vi "Acquire Data_RT.vi"(7 "Total Buffer Size":i32, 8 "error in (no error)":errorcluster, 9 "rt fifo":refnum<k33>, 10 "Acquisition and Logging Configuration":T1={"Data Rate"=1, "Samples per Read"=0, "Number of Reads to Save"=0, "Data File Name"="", "TDMS Properties"=[], "Number of Channels"=4, "Channel Scale Array"=[0.0, 0.0, 0.0, 0.0, 1.0, 1.0, 1.0, 1.0], "Channel Names"=[], "Trigger - RMS Value"=0.0, "Trigger - Channel"=0, "Trigger - Time (Minute)"=0} {"Data Rate" items=["51.200 kS/s (NI 9234)"=1, "25.600 kS/s (NI 9234)"=2, "17.067 kS/s (NI 9234)"=3, "12.800 kS/s (NI 9234)"=4, "10.240 kS/s (NI 9234)"=5, "8.533 kS/s (NI 9234)"=6, "7.314 kS/s (NI 9234)"=7, "6.400 kS/s (NI 9234)"=8, "5.689 kS/s (NI 9234)"=9, "5.120 kS/s (NI 9234)"=10, "4.654 kS/s (NI 9234)"=11, "4.267 kS/s (NI 9234)"=12, "3.938 kS/s (NI 9234)"=13, "3.657 kS/s (NI 9234)"=14, "3.413 kS/s (NI 9234)"=15, "3.200 kS/s (NI 9234)"=16, "3.012 kS/s (NI 9234)"=17, "2.845 kS/s (NI 9234)"=18, "2.695 kS/s (NI 9234)"=19, "2.560 kS/s (NI 9234)"=20, "2.438 kS/s (NI 9234)"=21, "2.328 kS/s (NI 9234)"=22, "2.226 kS/s (NI 9234)"=23, "2.133 kS/s (NI 9234)"=24, "2.048 kS/s (NI 9234)"=25, "1.969 kS/s (NI 9234)"=26, "1.896 kS/s (NI 9234)"=27, "1.829 kS/s (NI 9234)"=28, "1.765 kS/s (NI 9234)"=29, "1.707 kS/s (NI 9234)"=30, "1.652 kS/s (NI 9234)"=31]}, 11 "FPGA VI Reference":T4) -> (0 "error out":errorcluster, 2 "dup Acquisition and Logging Configuration":T1={"Data Rate"=1, "Samples per Read"=0, "Number of Reads to Save"=0, "Data File Name"="", "TDMS Properties"=[], "Number of Channels"=4, "Channel Scale Array"=[0.0, 0.0, 0.0, 0.0, 1.0, 1.0, 1.0, 1.0], "Channel Names"=[], "Trigger - RMS Value"=0.0, "Trigger - Channel"=0, "Trigger - Time (Minute)"=0} {"Data Rate" items=["51.200 kS/s (NI 9234)"=1, "25.600 kS/s (NI 9234)"=2, "17.067 kS/s (NI 9234)"=3, "12.800 kS/s (NI 9234)"=4, "10.240 kS/s (NI 9234)"=5, "8.533 kS/s (NI 9234)"=6, "7.314 kS/s (NI 9234)"=7, "6.400 kS/s (NI 9234)"=8, "5.689 kS/s (NI 9234)"=9, "5.120 kS/s (NI 9234)"=10, "4.654 kS/s (NI 9234)"=11, "4.267 kS/s (NI 9234)"=12, "3.938 kS/s (NI 9234)"=13, "3.657 kS/s (NI 9234)"=14, "3.413 kS/s (NI 9234)"=15, "3.200 kS/s (NI 9234)"=16, "3.012 kS/s (NI 9234)"=17, "2.845 kS/s (NI 9234)"=18, "2.695 kS/s (NI 9234)"=19, "2.560 kS/s (NI 9234)"=20, "2.438 kS/s (NI 9234)"=21, "2.328 kS/s (NI 9234)"=22, "2.226 kS/s (NI 9234)"=23, "2.133 kS/s (NI 9234)"=24, "2.048 kS/s (NI 9234)"=25, "1.969 kS/s (NI 9234)"=26, "1.896 kS/s (NI 9234)"=27, "1.829 kS/s (NI 9234)"=28, "1.765 kS/s (NI 9234)"=29, "1.707 kS/s (NI 9234)"=30, "1.652 kS/s (NI 9234)"=31]}, 3 "rt fifo out":refnum<k33>)   [LabVIEW 2015]
doc: "Reads waveform data from the DMA FIFO."
uses:
  controls/FPGA VI Reference.ctl
  controls/Acquisition and Logging Configuration.ctl
  <vilib>/LabVIEW Targets/FPGA/cRIO/shared/nicrio_ModuleControls/nicrio_cRIO-9234_DataRatesRing2.ctl
  controls/TDMS Properties.ctl
  <vilib>/Platform/TimedLoop/XDataNode/timing_clust.ctl
  <vilib>/Platform/TimedLoop/XDataNode/nitl_modes.ctl
  <vilib>/Platform/TimedLoop/XDataNode/wakeup.ctl
  <vilib>/Utility/error.llb/Error Cluster From Error Code.vi
  <vilib>/rvi/errors/niLvFpgaAdjustHostInterfaceError.vi
  Globals/Global - Monitoring Variables.vi
  <vilib>/rvi/interface/nirviReadWriteControl/nirviReadWriteControl.xnode
  <vilib>/rvi/interface/nirviMethod/nirviMethod.xnode
  <vilib>/Platform/TimedLoop/XDataNode/XDataNode.xnode
  NiFpgaLv.dll
  <vilib>/rvi/interface/Simulation/niFpgaSimulationCallBeginRW.vi
  <vilib>/FPGAPlugInAG/Dynamic/niLvFpga_ReadFifo_Dynamic.vi
  <vilib>/rvi/errors/niLvFpgaMergeErrorWithErrorCode.vi
  <vilib>/Platform/TimedLoop/XDataNode/XDNodeRunTimeDep.lvlib
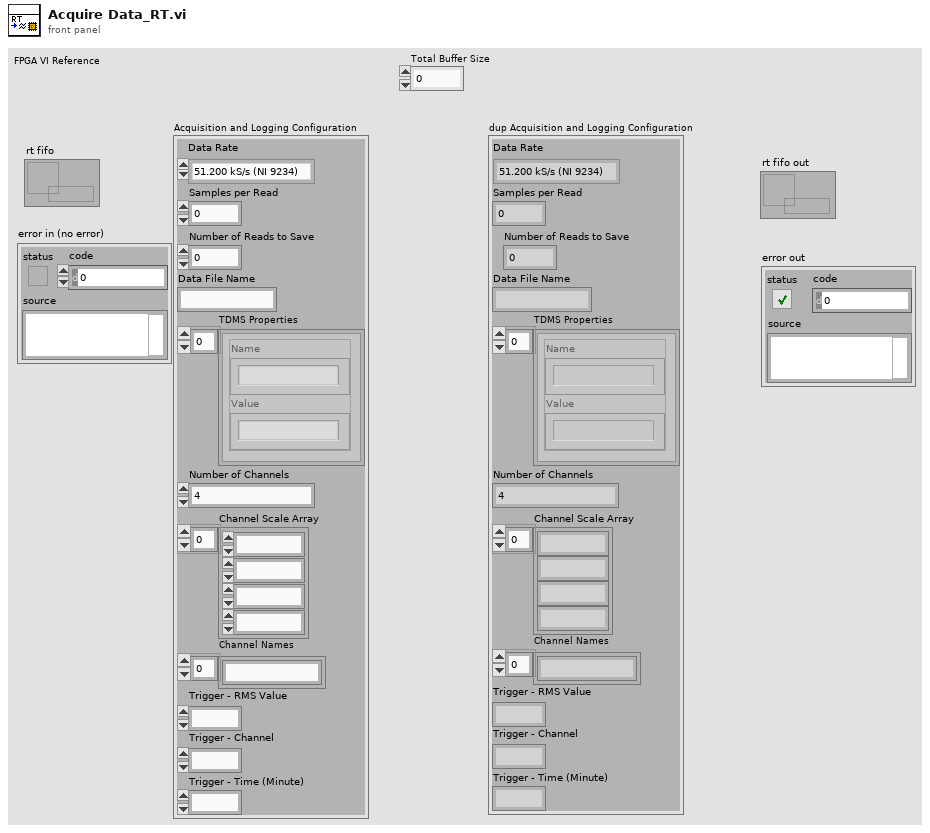
[diagram p1: front panel]
types:
  T1 = typedef "Acquisition and Logging Configuration.ctl" = cluster{"Data Rate":T2, "Samples per Read":i32, "Number of Reads to Save":i32, "Data File Name":string, "TDMS Properties":T3[], "Number of Channels":i32, "Channel Scale Array":fxp<+,24,12>[], "Channel Names":string[], "Trigger - RMS Value":dbl, "Trigger - Channel":i32, "Trigger - Time (Minute)":i32}
  T2 = typedef "nicrio_cRIO-9234_DataRatesRing2.ctl" = u8
  T3 = typedef "TDMS Properties.ctl" = cluster{"Name":string, "Value":string}
  T4 = typedef "FPGA VI Reference.ctl" = refnum<k20>
  T5 = typedef "XDNodeRunTimeDep.lvlib/timing_clust.ctl" = cluster{"Expected End [f-1]":u64, "Actual End [f-1]":u64, "Finished Late? [f-1]":bool, "Expected End [i-1]":u64, "Actual End [i-1]":u64, "Finished Late? [i-1]":bool, "Expected Start [i]":u64, "Actual Start [i]":u64, "Expected Start [f]":u64, "Actual Start [f]":u64, "Source Name":string, "Structure Name":string, "Period":i64, "Deadline":i64, "Offset":i64, "Start":i64, "Priority":i32, "Timeout":i32, "Mode":T6, "Wakeup Reason":T7, "Error":errorcluster, "Source Type":string, "Secondary Source Type":string, "Global End Time":u64, "Global Start Time":u64, "Frame Duration":u64, "Iteration Duration":u64, "Assigned CPU":i32, "I/O Scan Engine Mode":u32}
  T6 = typedef "XDNodeRunTimeDep.lvlib/nitl_modes.ctl" = enum32{"No Change", "Process missed periods, maintain original phase", "Discard missed periods, maintain original phase", "Process missed periods, ignore original phase", "Discard missed periods, ignore original phase"}
  T7 = typedef "XDNodeRunTimeDep.lvlib/wakeup.ctl" = enum32{"Normal", "Aborted", "Asynchronous wakeup", "Timing source error", "Timed loop error", "Timeout"}
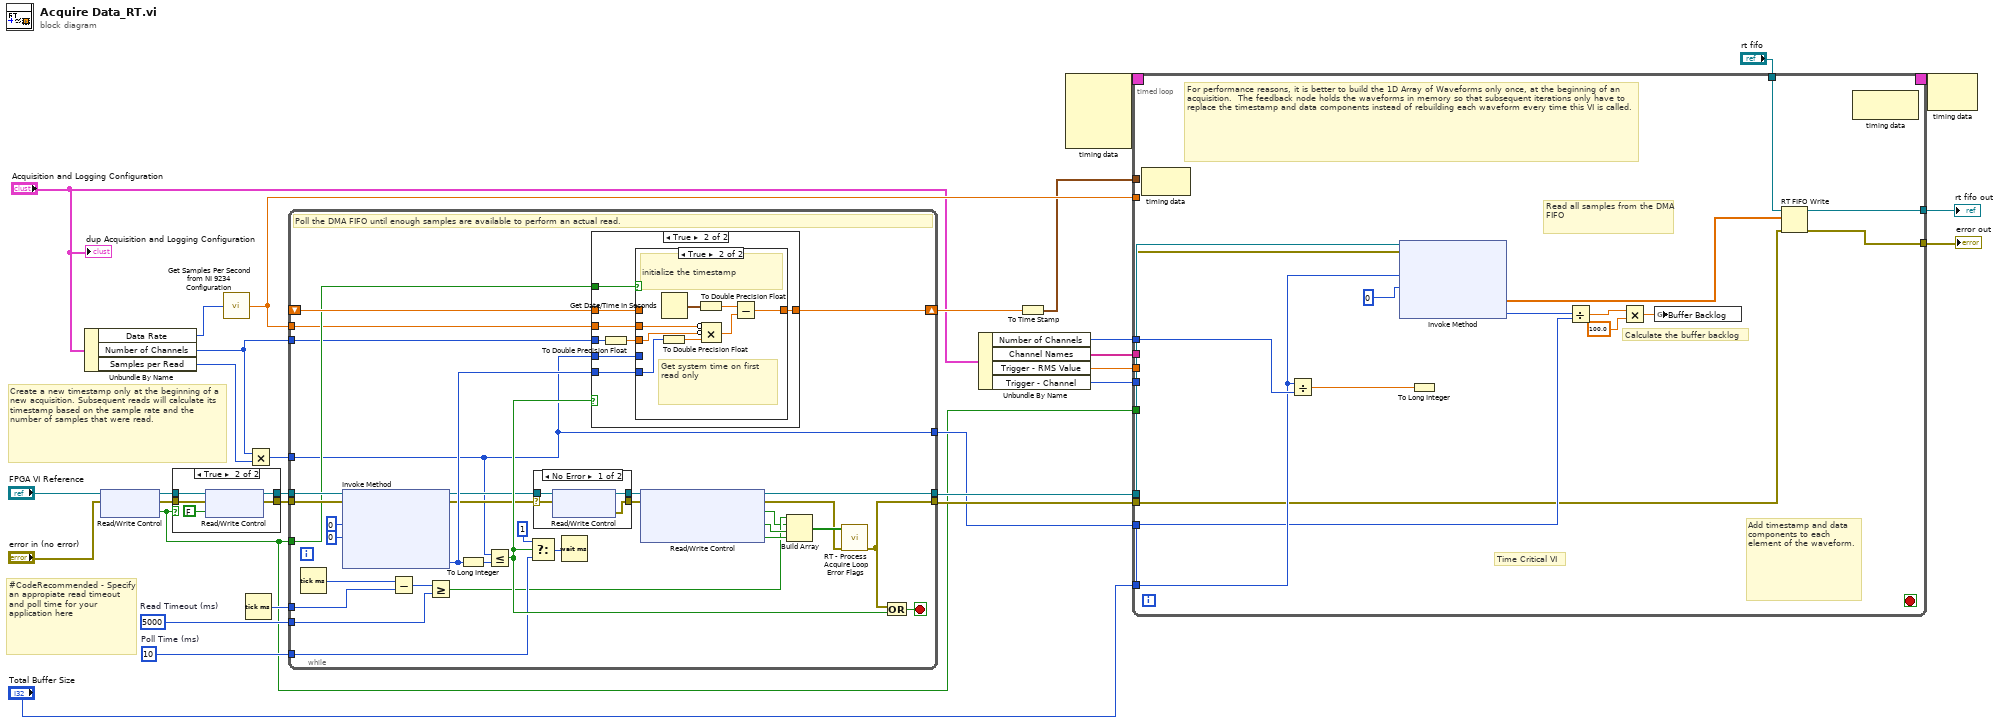
[diagram p0: block diagram]
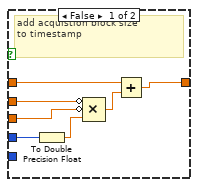
[diagram p4: hidden frame]
diagram:
  w14 = u32 10  # Poll Time (ms)
  w15 = u32 5000  # Read Timeout (ms)
  # "#CodeRecommended - Specify an appropiate read timeout and poll time for your application here"
  # "Create a new timestamp only at the beginning of a new acquisition. Subsequent reads will calculate its timestamp based on the sample rate and the number of samples that were read."
  n1 = Unbundle By Name("Acquisition and Logging Configuration") -> ("Data Rate"=w8:T2, "Number of Channels"=w6:i32, "Samples per Read"=w7:i32)
  n2 = xnode "Read/Write Control"("FPGA VI Reference In"="FPGA VI Reference", "error in"="error in (no error)") -> ("FPGA VI Reference Out"=w29:T4, "error out"=w30:errorcluster, "First Read"=w11:bool)
  n3 = case shown="True" w11 {
    tunnel: w29 -> [w33 w38]
    tunnel: [w33 w37] -> w27
    tunnel: w30 -> [w32 w36]
    tunnel: [w32 w35] -> w26
    frame False {
    }
    frame True {
      n4 = xnode "Read/Write Control"("FPGA VI Reference In"=w38, "error in"=w36, "First Read"=FALSE) -> ("FPGA VI Reference Out"=w37:T4, "error out"=w35:errorcluster)
    }
  }
  n5 = call "Get Samples Per Second from NI 9234 Configuration.vi"("Sample Rate (51.2k )"=w8) -> ("Samples per second"=w31:dbl)  [unwired: 4 in]
  n6 = Tick Count (ms)() -> (millisecond timer value=w25:u32)
  n7 = Multiply(x=w6, y=w7) -> (x*y=w18:i32)
  n8 = while {
    tunnel: [w43] -> w23
    tunnel: [w49] -> w24
    tunnel: w11 -> [w66]
    tunnel: w27 -> [w69]
    tunnel: w26 -> [w68]
    shift-right: [w61] -> w21
    shift-left: _ -> [w67]
    tunnel: w25 -> [w70]
    tunnel: w18 -> [w39]
    tunnel: [w39] -> w13
    tunnel: w6 -> [w40]
    tunnel: w15 -> [w55]
    tunnel: w14 -> [w54]
    tunnel: w31 -> [w41]
    stop <- w71 stop-if-true
    # "Poll the DMA FIFO until enough samples are available to perform an actual read."
    n9 = Tick Count (ms)() -> (millisecond timer value=w65:u32)
    n10 = xnode "Invoke Method"("FPGA VI Reference In"=w69, "error in"=w68, "Number of Elements"=u32 0, "Timeout (ms)"=0) -> ("FPGA VI Reference Out"=w52:T4, "error out"=w53:errorcluster, "Elements Remaining"=w57:u32)  [unwired: 1 out]
    n11 = Subtract(x=w65, y=w70) -> (x-y=w56:u32)
    n12 = Greater Or Equal?(x=w56, y=w55) -> (x >= y?=w46:bool)
    n13 = To Long Integer(number=w57) -> (32bit integer=w60:i32)
    n14 = Less Or Equal?(x=w39, y=w60) -> (x <= y?=w64:bool)
    n15 = Select(t=u32 1, s=w64, f=w54) -> (s? t:f=w63:u32)
    n16 = case shown="No Error" w53 {
      selector: w53 -> [w75 w76]
      tunnel: w52 -> [w74 w77]
      tunnel: [w73 w77] -> w51
      tunnel: [w72 w76] -> w50
      frame No Error {
        n17 = xnode "Read/Write Control"("FPGA VI Reference In"=w74, "error in"=w75) -> ("FPGA VI Reference Out"=w73:T4, "FPGA Error"=w72:errorcluster)  [unwired: 1 out]
      }
      frame Error {
      }
    }
    n18 = Wait (ms)(milliseconds to wait=w63) -> ()  [unwired: 1 out]
    n19 = case shown="True" w64 {
      tunnel: w67 -> [w78 w86]
      tunnel: w66 -> [_ w85]
      tunnel: w57 -> [_ w84]
      tunnel: [w78 w83] -> w61
      tunnel: w39 -> [_ w82]
      tunnel: w41 -> [_ w80]
      tunnel: w40 -> [_ w79]
      frame False {
      }
      frame True {
        n20 = To Double Precision Float(number=w79) -> (double precision float=w81:dbl)
        n21 = case shown="True" w85 {
          tunnel: w80 -> [w91 w101]
          tunnel: w86 -> [w92 _]
          tunnel: w82 -> [w88 _]
          tunnel: w81 -> [w89 w100]
          tunnel: w84 -> [_ w95]
          tunnel: [w93 w97] -> w83
          frame False {
            # "add acquistion block size\nto timestamp"
            n22 = To Double Precision Float(number=w88) -> (double precision float=w87:dbl)
            n23 = Compound Arithmetic op=MULTIPLY(invert w91, invert w89, w87) -> (w90:dbl)
            n24 = Add(x=w92, y=w90) -> (x+y=w93:dbl)
          }
          frame True {
            # "Get system time on first read only"
            # "initialize the timestamp"
            n25 = To Double Precision Float(number=w95) -> (double precision float=w94:dbl)
            n26 = Get Date/Time In Seconds() -> (seconds since 1Jan1904=w99:timestamp)
            n27 = To Double Precision Float(number=w99) -> (double precision float=w96:dbl)
            n28 = Compound Arithmetic op=MULTIPLY(invert w101, invert w100, w94) -> (w98:dbl)
            n29 = Subtract(x=w96, y=w98) -> (x-y=w97:dbl)
          }
        }
      }
    }
    n30 = xnode "Read/Write Control"("FPGA VI Reference In"=w51, "error in"=w50) -> ("FPGA VI Reference Out"=w49:T4, "error out"=w42:errorcluster, "Module Underflow"=w45:bool, "DMA FIFO Full"=w48:bool, "Different Channel Count"=w47:bool)
    n31 = Build Array(w46, w45, w48, w47) -> (w44:bool[])
    n32 = call "RT - Process Acquire Loop Error Flags.vi"("error in (no error)"=w42, "Error Flags"=w44) -> ("error out"=w43:errorcluster)  [unwired: 9 in]
    n33 = Compound Arithmetic op=OR(w43, w64) -> (w71:bool)
  }
  n34 = Unbundle By Name("Acquisition and Logging Configuration") -> ("Number of Channels"=w17:i32, "Channel Names"=w19:string[], "Trigger - RMS Value"=w20:dbl, "Trigger - Channel"=w22:i32)
  n35 = To Time Stamp(1:w21) -> (0:w12:timestamp)
  n36 = node-c288() -> (w5:T5)  [unwired: 4 in]
  n37 = timed-loop {
    timing: w5 -> [_]
    timing-out: [_] -> w4
    tunnel: w31 -> [_]
    tunnel: w24 -> [w116]
    tunnel: w23 -> [w103]
    tunnel: w22 -> [_]
    tunnel: w20 -> [_]
    tunnel: w19 -> [_]
    tunnel: w17 -> [w115]
    tunnel: w13 -> [w113]
    tunnel: w12 -> [_]
    tunnel: w11 -> [_]
    tunnel: "Total Buffer Size" -> [w108]
    tunnel: [w106] -> w3
    tunnel: "rt fifo" -> [w105]
    tunnel: [w102] -> w1
    stop <- _ stop-if-true
    # "Time Critical VI"
    # "Calculate the buffer backlog"
    # "For performance reasons, it is better to build the 1D Array of Waveforms only once, at the beginning of an acquisition.  The feedback node holds the waveforms in memory so that subsequent iterations only have to replace the timestamp and data components instead of rebuilding each waveform every time this VI is called."
    # "Read all samples from the DMA FIFO"
    # "Add timestamp and data components to each element of the waveform."
    n38 = node-c288() -> ()  [unwired: 1 in, 1 out]
    n39 = Divide(x=w113, y=w115) -> (x/y=w114:dbl)
    n40 = xnode "Invoke Method"("FPGA VI Reference In"=w116, "error in"=w103, "Number of Elements"=w113, "Timeout (ms)"=0) -> ("Data"=w104:sgl[], "Elements Remaining"=w111:u32)  [unwired: 2 out]
    n41 = To Long Integer(number=w114) -> ()  [unwired: 1 out]
    n42 = Divide(x=w111, y=w108) -> (x/y=w112:dbl)
    n43 = Multiply(x=w112, y=100.0) -> (x*y=w109:dbl)
    n44 = global write "Global - Monitoring Variables.vi" "Buffer Backlog"(w109) -> ()
    n45 = RT FIFO Write(0:w105, 1:w104, 3:w103) -> (8:w106:refnum<k33>, 11:w102:errorcluster)  [unwired: 2 in, 2 out]
    n46 = node-c288() -> ()  [unwired: 1 in, 1 out]
  }
  "rt fifo out" <- w3
  "error out" <- w1
  n47 = node-c288(w4) -> ()  [unwired: 1 out]
  "dup Acquisition and Logging Configuration" <- "Acquisition and Logging Configuration"
